vi "GE 5565PIORC.VISA Resource Name.vi"() -> (3 "VISA resource name":refnum<visa-resource-name>)   [LabVIEW 2016]
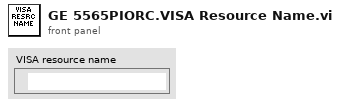
[diagram p1: front panel]
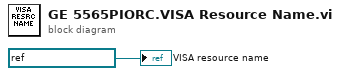
[diagram p0: block diagram]
diagram:
  "VISA resource name" <- refnum<visa-resource-name> "PXI4::14::INSTR" ("VISA resource name")
